vi "Read Direccion.vi"(8 "error in (no error)":errorcluster, 11 "Logging_txt in":refnum<class "Logging_txt.lvclass">) -> (0 "error out":errorcluster, 2 "Direccion":path, 3 "Logging_txt out":refnum<class "Logging_txt.lvclass">)   [LabVIEW 2019, in "Logging_txt.lvlib" / "Logging_txt.lvclass"]
uses:
  Logging_txt.lvclass
  Logging_txt.lvclass/Logging_txt.ctl
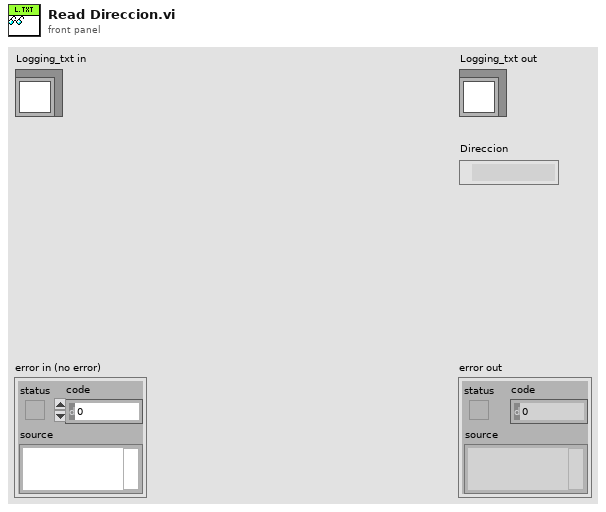
[diagram p1: front panel]
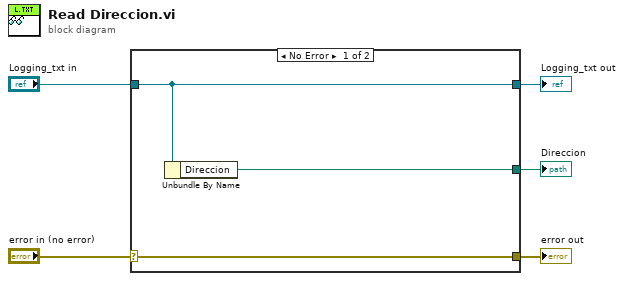
[diagram p0: block diagram]
diagram:
  n1 = case shown="No Error" "error in (no error)" {
    selector: "error in (no error)" -> [w8 w9]
    tunnel: [w8 w9] -> w4
    tunnel: [w7 w10] -> w2
    tunnel: "Logging_txt in" -> [w7 w10]
    tunnel: [w6 _] -> w1
    frame No Error {
      n2 = Unbundle By Name(w7) -> ("Direccion"=w6:path)
    }
    frame Error {
    }
  }
  "error out" <- w4
  "Logging_txt out" <- w2
  "Direccion" <- w1
